vi "_PC_SaveFile FilePathFGV.vi"(10 "Reload? (F)":bool, 11 "TreeControl in":refnum<vi>) -> (2 "Numeric":i32, 3 "datas path":path[](array[path]))   [LabVIEW 2018]
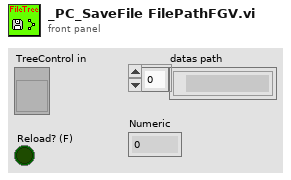
[diagram p1: front panel]
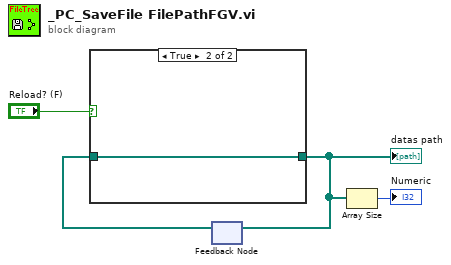
[diagram p0: block diagram]
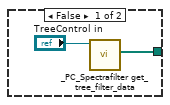
[diagram p2: hidden frame]
diagram:
  n1 = feedback #1() -> (w2:path[])  [unwired: 1 in]
  n2 = case shown="True" "Reload? (F)" {
    tunnel: [w5 w7] -> w3
    tunnel: w2 -> [_ w7]
    frame False {
      n3 = call "_PC_Spectrafilter get_tree_filter_data.vi"("file tree ref"="TreeControl in") -> ("datas path"=w5:path[])  [unwired: 9 in, 1 out]
    }
    frame True {
    }
  }
  "datas path" <- w3
  n4 = feedback-in #1(w3) -> ()
  n5 = Array Size(array=w3) -> (size(s)=→"Numeric":i32)
